vi "PowerMonitor.vi"() -> ()   [LabVIEW 2013]
panel:
  out "data":dbl
  out "podglad":dynamicdata(graph)
  in  "stop":bool
  # "Podgląd mocy detekowanej wiązki:"
  # "Detekowana wartość:"
  # "Zatrzymaj działanie programu, aby wrócić do panelu pomiarowego"
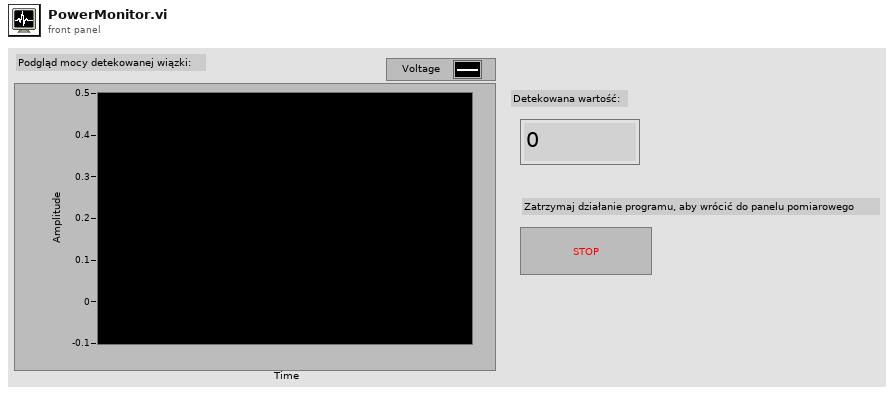
[diagram p1: front panel]
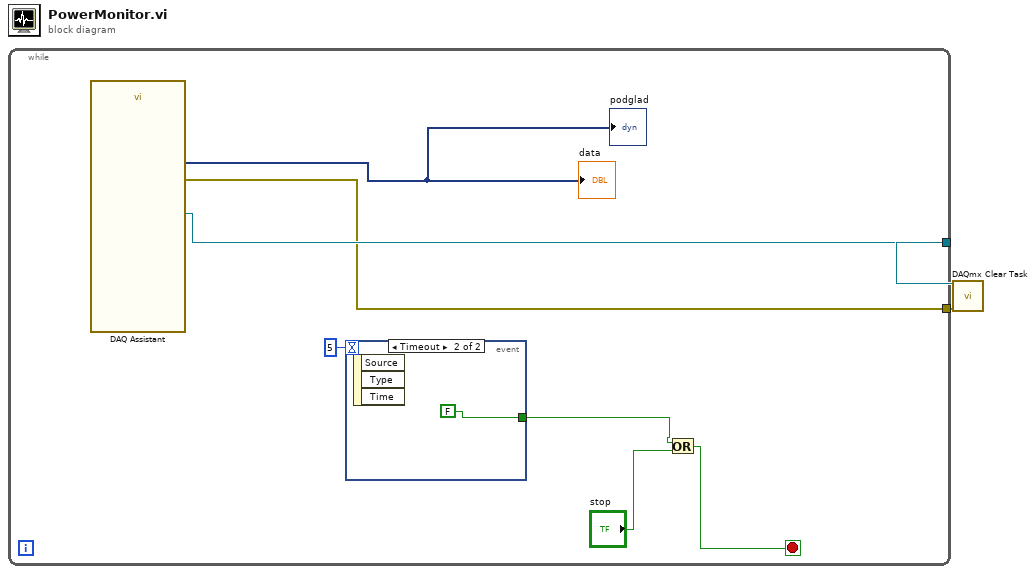
[diagram p0: block diagram]
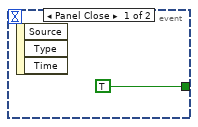
[diagram p2: hidden frame]
diagram:
  n1 = while {
    tunnel: [w4] -> w2
    tunnel: [w3] -> w1
    stop <- w6 stop-if-true
    n2 = call "DAQ Assistant"() -> ("task out"=w4:refnum<k21>, "data"=→"podglad" →"data":dynamicdata, "error out"=w3:errorcluster)  [unwired: 16 in, 1 out]
    n3 = event shown="[1] Timeout" {
      selector: _ -> [_ _]
      dyn-events: _ -> [_ _]
      timeout: 5 -> [_ _]
      tunnel: [TRUE FALSE] -> w9
      event Panel Close {
        n4 = event-data() -> ()  [unwired: 1 in, 3 out]
      }
      event Timeout {
        n5 = event-data() -> ()  [unwired: 1 in, 3 out]
      }
    }
    n6 = Or(x=w9, y="stop") -> (x .or. y?=w6:bool)
  }
  n7 = call <vilib>:"DAQmx Clear Task.vi"("task in"=w2, "error in"=w1) -> ()  [unwired: 13 in, 1 out]
